vi "practiceImageAnalysis.vi"() -> ()   [LabVIEW 2016]
panel:
  out "Images Array":T1[](array[plugin-control])
  in  "error in":errorcluster
  out "error out":errorcluster
  out "Filenames Array":string[](array[string])
  in  "Naming Convention":string="*.png"
  in  "Images Directory":path=path "E:/XYZstage+Camera_CollectedImages/12-16-2016/noStaveMount/toolingpins_images"
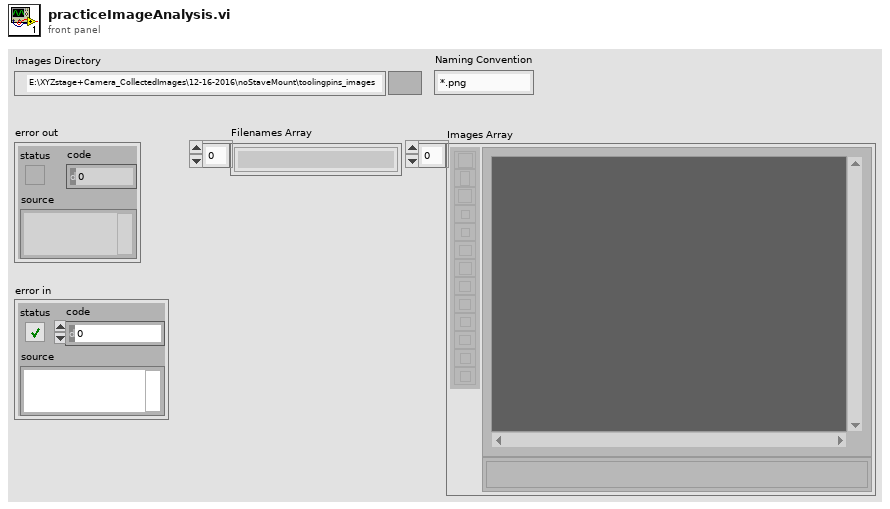
[diagram p1: front panel]
types:
  T1 = typedef "IMAQ Image.ctl" = refnum<image>
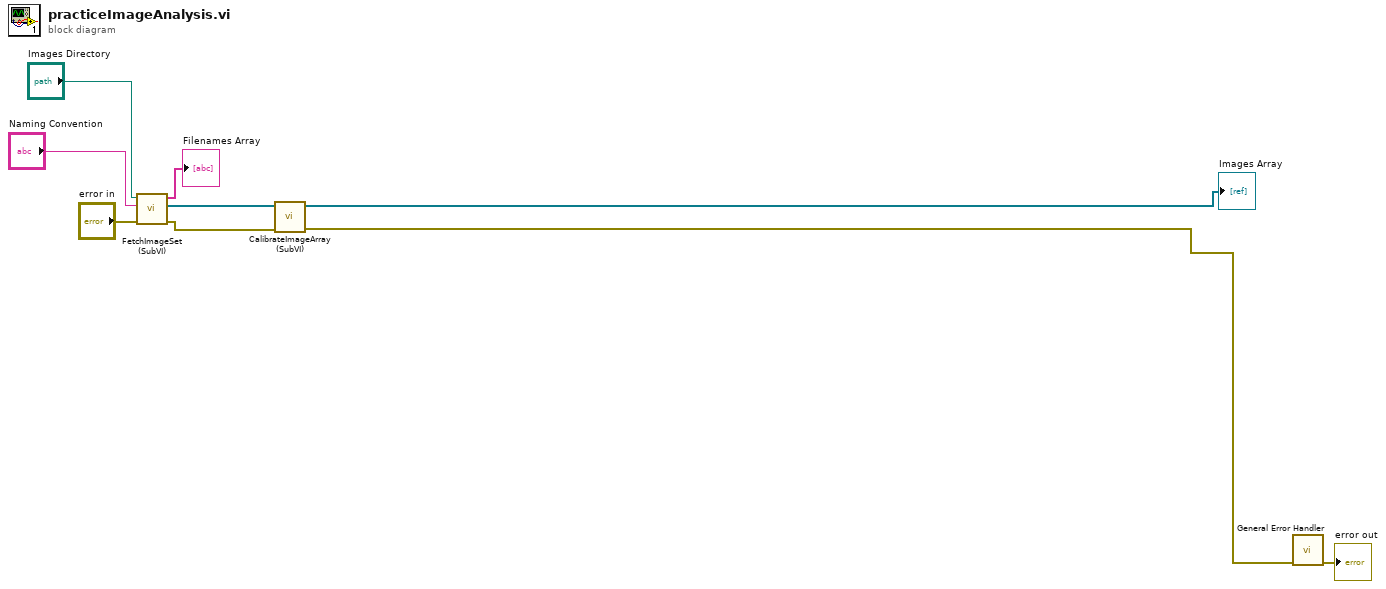
[diagram p0: block diagram]
diagram:
  n1 = call "FetchImageSet (SubVI).vi"("error in (no error)"="error in", "Naming Convention"="Naming Convention", "Images Directory"="Images Directory") -> ("error out"=w4:errorcluster, "Image Array"=w5:T1[], "Filenames Array"=→"Filenames Array":string[])  [unwired: 6 in]
  n2 = call "CalibrateImageArray (SubVI).vi"("error in (no error)"=w4, "Image Array"=w5) -> ("error out"=w1:errorcluster, "Calibrated Image Array"=→"Images Array":T1[])  [unwired: 7 in]
  n3 = call <vilib>:"General Error Handler.vi"("error in (no error)"=w1) -> ("error out"=→"error out":errorcluster)  [unwired: 10 in, 4 out]
